vi "Add Parameter Channels for SDI SSM Parity.vi"(8 "error in":errorcluster, 10 "label name":string, 11 "label parameters":T4) -> (0 "error out":errorcluster, 3 "parameters in word":T1[](array[typedef]))   [LabVIEW 2020, in "Communication Bus Template Scripting.lvlib"]
uses:
  Communication Bus Template Scripting.lvlib
  ARINC 429 Channel Definition.ctl
  Channel Parameter.ctl
  Protocol/Implementations/ARINC429/Parameter Definition.ctl
  Encoding and Decoding/Encoding.ctl
  Protocol/Implementations/ARINC429/ARINC 429.lvclass
  Encoding and Decoding/Encoding and Decoding.lvlib
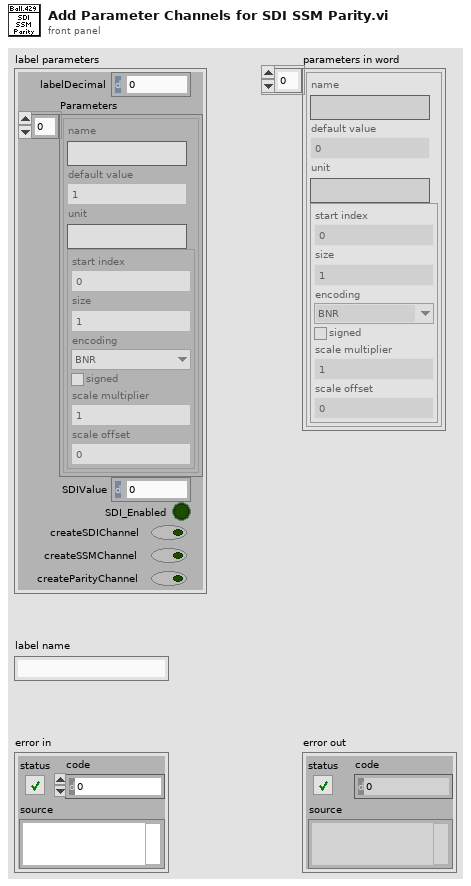
[diagram p1: front panel]
types:
  T1 = typedef "Communication Bus Template Scripting.lvlib/Channel Parameter.ctl" = cluster{"name":string, "default value":dbl, "unit":string, "Parameter":T2}
  T2 = typedef "ARINC 429.lvclass/Parameter Definition.ctl" = cluster{"start index":i32, "size":i32, "encoding":T3, "signed":bool, "scale multiplier":dbl, "scale offset":dbl}
  T3 = typedef "Encoding and Decoding.lvlib/Encoding.ctl" = enum16{"BNR", "BCD", "Discrete"}
  T4 = typedef "Communication Bus Template Scripting.lvlib/ARINC 429 Channel Definition.ctl" = cluster{"labelDecimal":i32, "Parameters":T1[], "SDIValue":u8, "SDI_Enabled":bool, "createSDIChannel":bool, "createSSMChannel":bool, "createParityChannel":bool}
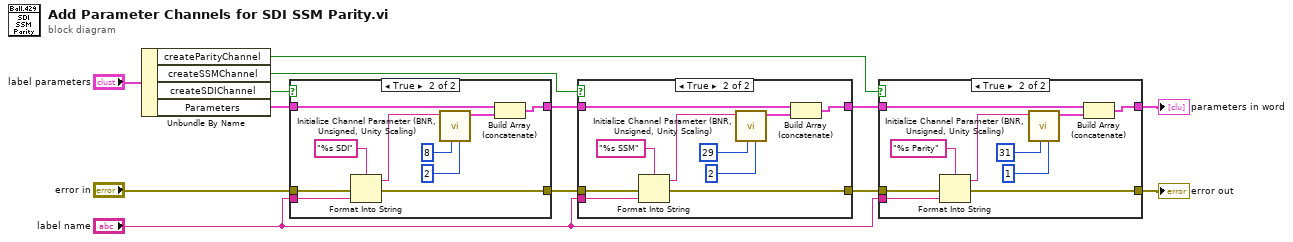
[diagram p0: block diagram]
diagram:
  n1 = Unbundle By Name("label parameters") -> ("createParityChannel"=w2:bool, "createSSMChannel"=w3:bool, "createSDIChannel"=w13:bool, "Parameters"=w1:T1[])
  n2 = case shown="True" w13 {
    tunnel: w1 -> [w15 w25]
    tunnel: [w15 w24] -> w11
    tunnel: "label name" -> [_ w23]
    tunnel: "error in" -> [w14 w21]
    tunnel: [w14 w20] -> w10
    frame False {
    }
    frame True {
      n3 = Format Into String(format string="%s SDI", error in=w21, w23) -> (resulting string=w19:string, error out=w20:errorcluster)  [unwired: 1 in]
      n4 = call "Initialize Channel Parameter (BNR, Unsigned, Unity Scaling).vi"("size"=2 ("numberOfBits"), "start index"=8 ("startBit"), "name"=w19) -> ("channel parameter"=w18:T1)  [unwired: 8 in]
      n5 = Build Array (concatenate)(w25, w18) -> (w24:T1[])
    }
  }
  n6 = case shown="True" w3 {
    tunnel: [w26 w37] -> w6
    tunnel: "label name" -> [_ w36]
    tunnel: w10 -> [w27 w34]
    tunnel: [w27 w33] -> w9
    tunnel: w11 -> [w26 w32]
    frame False {
    }
    frame True {
      n7 = Format Into String(format string="%s SSM", error in=w34, w36) -> (resulting string=w31:string, error out=w33:errorcluster)  [unwired: 1 in]
      n8 = call "Initialize Channel Parameter (BNR, Unsigned, Unity Scaling).vi"("size"=2 ("numberOfBits"), "start index"=29 ("startBit"), "name"=w31) -> ("channel parameter"=w30:T1)  [unwired: 8 in]
      n9 = Build Array (concatenate)(w32, w30) -> (w37:T1[])
    }
  }
  n10 = case shown="True" w2 {
    tunnel: "label name" -> [_ w49]
    tunnel: w9 -> [w39 w47]
    tunnel: [w39 w46] -> w7
    tunnel: w6 -> [w38 w45]
    tunnel: [w38 w44] -> w5
    frame False {
    }
    frame True {
      n11 = Format Into String(format string="%s Parity", error in=w47, w49) -> (resulting string=w43:string, error out=w46:errorcluster)  [unwired: 1 in]
      n12 = call "Initialize Channel Parameter (BNR, Unsigned, Unity Scaling).vi"("size"=1 ("numberOfBits"), "start index"=31 ("startBit"), "name"=w43) -> ("channel parameter"=w42:T1)  [unwired: 8 in]
      n13 = Build Array (concatenate)(w45, w42) -> (w44:T1[])
    }
  }
  "error out" <- w7
  "parameters in word" <- w5
